vi "CRYRead Config Settings Key.vi"(10 "Key Names":string[](array[string]), 11 "Items":cluster{"Key":string, "Value":string}[](array[cluster])) -> (2 "Values":string[](array[string]))   [LabVIEW 2013]
doc: "Illustrates how to read a configuration settings file.\n\nInstructions:\nRun Write Configuration Settings File.vi, located in the file\\config.llb. Then run this VI and select the appropriate configuration settings file to load."
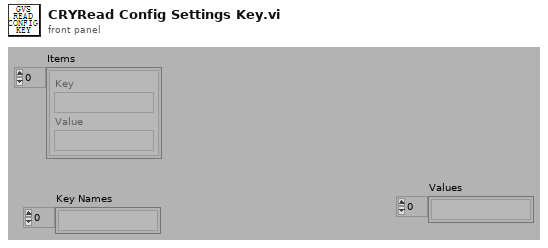
[diagram p1: front panel]
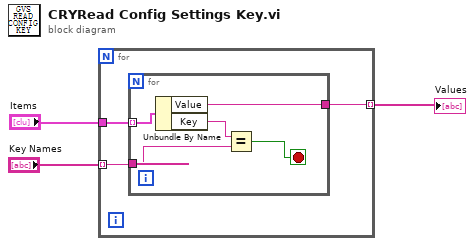
[diagram p0: block diagram]
diagram:
  n1 = for {
    tunnel: "Key Names" -> [w6] mode=indexing
    tunnel: "Items" -> [w5]
    tunnel: [w4] -> w1 mode=indexing
    n2 = for {
      tunnel: w6 -> [w9]
      tunnel: w5 -> [w11] mode=indexing
      tunnel: [w7] -> w4
      stop <- w8 stop-if-true
      n3 = Unbundle By Name(w11) -> ("Value"=w7:string, "Key"=w10:string)
      n4 = Equal?(x=w10, y=w9) -> (x = y?=w8:bool)
    }
  }
  "Values" <- w1
